vi "Check Ordered Hash.vi"(8 "error in":errorcluster, 11 "refnum":T2) -> (0 "error out":errorcluster, 1 "Key":string, 2 "Canceled?":bool, 3 "refnum out":T2, 4 "Sorted Data":T1)   [LabVIEW 2013]
uses:
  <vilib>/Utility/config.llb/Config Data RefNum.ctl
  <vilib>/Utility/config.llb/NI_LVConfig.lvlib
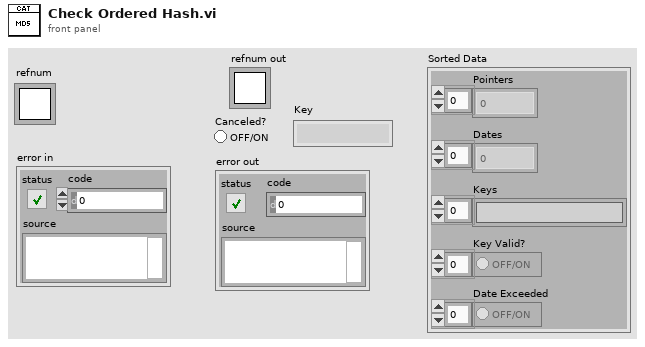
[diagram p1: front panel]
types:
  T1 = cluster{"Pointers":i32[], "Dates":dbl[], "Keys":string[], "Key Valid?":bool[], "Date Exceeded":bool[]}
  T2 = typedef "NI_LVConfig.lvlib/Config Data RefNum.ctl" = refnum<k1>
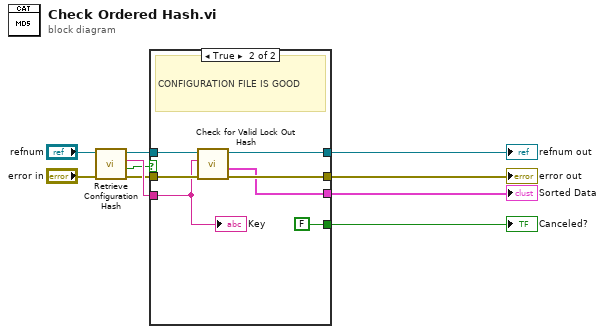
[diagram p0: block diagram]
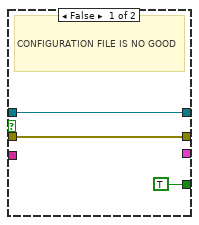
[diagram p2: hidden frame]
diagram:
  n1 = call "Retrieve Configuration Hash.vi"("error in"="error in", "Refnum in"="refnum") -> ("error out"=w3:errorcluster, "Hash Good?"=w2:bool, "Key Out"=w5:string, "Refnum out"=w4:T2)  [unwired: 6 in]
  n2 = case shown="True" w2 {
    tunnel: [TRUE ("Canceled?") FALSE ("Canceled?")] -> w10
    tunnel: w3 -> [w12 w18]
    tunnel: w4 -> [w13 w17]
    tunnel: w5 -> [_ w16]
    tunnel: [w13 w20] -> w7
    tunnel: [w12 w19] -> w6
    tunnel: [_ w15] -> w1
    frame False {
      # "CONFIGURATION FILE IS NO GOOD"
    }
    frame True {
      # "CONFIGURATION FILE IS GOOD"
      n3 = call "Check for Valid Lock Out Hash.vi"("error in"=w18, "Key In"=w16, "Refnum in"=w17) -> ("error out"=w19:errorcluster, "Sorted Data"=w15:T1, "Refnum out"=w20:T2)  [unwired: 5 in, 1 out]
      "Key" <- w16
    }
  }
  "Canceled?" <- w10
  "refnum out" <- w7
  "error out" <- w6
  "Sorted Data" <- w1
